vi "doT1.vi"(8 "q_samples":i32=50, 10 "parameters_recenter":T5={"input_xyz"={"X_um"=0.0, "Y_um"=0.0, "Z_um"=0.0}, "recenter"=FALSE, "recenter_s"=3}, 11 "Rabi_parameters":T6) -> (0 "triggers":u32[][](array[numeric]), 1 "std_deviation":dbl[](array[numeric]), 2 "Rabi_curve":cluster{dbl[], "dark_time_us":dbl[]}(graph), 3 "timetags":u32[][](array[numeric]), 5 "position_xyzt":T1, 7 "mini_scan":T2)   [LabVIEW 2018]
uses:
  <vilib>/Analysis/NI_AALBase.lvlib
panel:
  in  "parameters_z-scan":T3={"dwell_time_ms"=2.0, "q_steps"=5, "span_um"=1.0, "refocus"=TRUE}
  in  "parameters_xy-scan":T4={"image_size_xy_um"=2.0, "frame_size_xy_px"=7, "dwell_time_ms"=0.5}
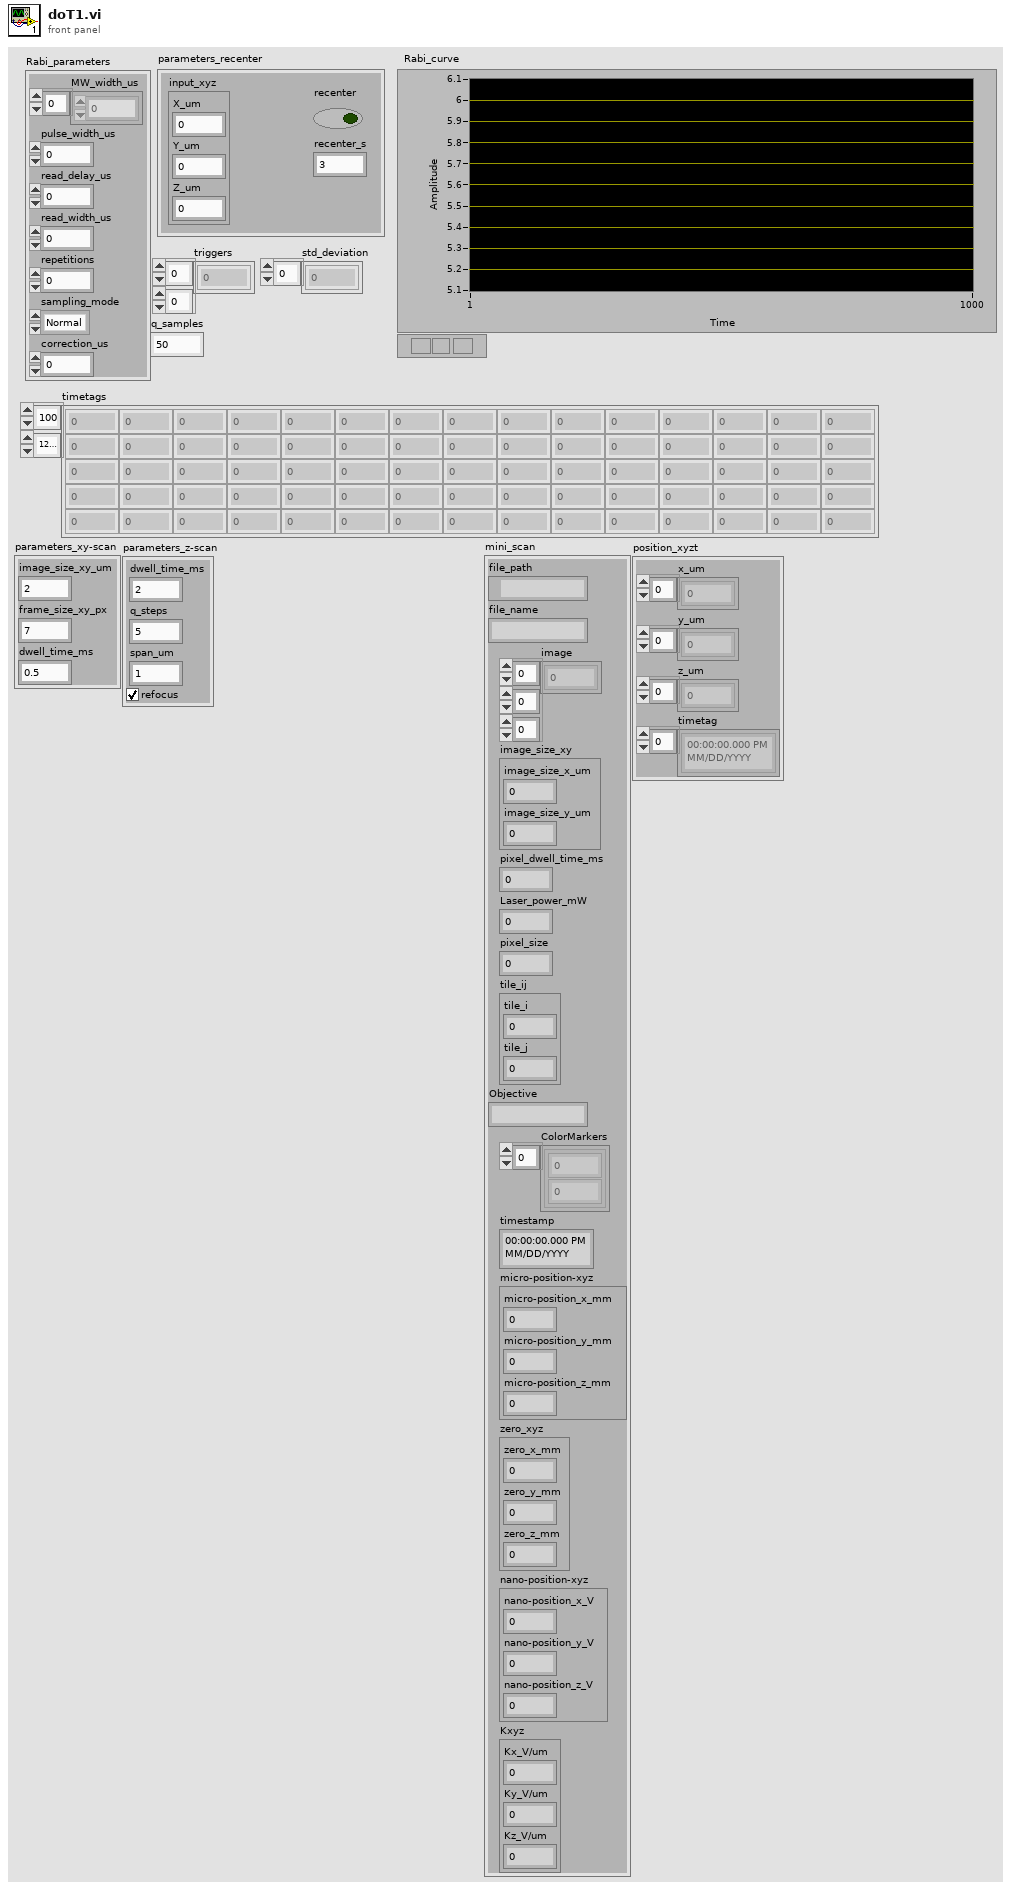
[diagram p1: front panel]
types:
  T1 = cluster{"x_um":sgl[], "y_um":sgl[], "z_um":sgl[], "timetag":timestamp[]}
  T2 = cluster{"file_path":path, "file_name":string, "image":dbl[][][], "image_size_xy":cluster{"image_size_x_um":sgl, "image_size_y_um":sgl}, "pixel_dwell_time_ms":sgl, "Laser_power_mW":sgl, "pixel_size":dbl, "tile_ij":cluster{"tile_i":i32, "tile_j":i32}, "Objective":string, "ColorMarkers":cluster{dbl, u32}[], "timestamp":timestamp, "micro-position-xyz":cluster{"micro-position_x_mm":sgl, "micro-position_y_mm":sgl, "micro-position_z_mm":sgl}, "zero_xyz":cluster{"zero_x_mm":dbl, "zero_y_mm":dbl, "zero_z_mm":dbl}, "nano-position-xyz":cluster{"nano-position_x_V":sgl, "nano-position_y_V":sgl, "nano-position_z_V":sgl}, "Kxyz":cluster{"Kx_V/um":sgl, "Ky_V/um":sgl, "Kz_V/um":sgl}}
  T3 = cluster{"dwell_time_ms":dbl, "q_steps":u32, "span_um":dbl, "refocus":bool}
  T4 = cluster{"image_size_xy_um":dbl, "frame_size_xy_px":u32, "dwell_time_ms":dbl}
  T5 = cluster{"input_xyz":cluster{"X_um":sgl, "Y_um":sgl, "Z_um":sgl}, "recenter":bool, "recenter_s":u32}
  T6 = cluster{"MW_width_us":dbl[], "pulse_width_us":dbl, "read_delay_us":dbl, "read_width_us":dbl, "repetitions":i32, "sampling_mode":enum16{"Normal", "Sweep"}, "correction_us":dbl}
  T7 = cluster{"Instruct Data":i32, "Op Code":i32, "Flags":bool[], "Comments":string, "Time":dbl}[]
  T8 = cluster{"nano-position_X_um":sgl, "nano-position_Y_um":sgl, "nano-position Z_um":sgl}
  T9 = cluster{"nano-position_X_um":sgl, "nano-position_Y_um":sgl, "nano-position Z_um":sgl}[]
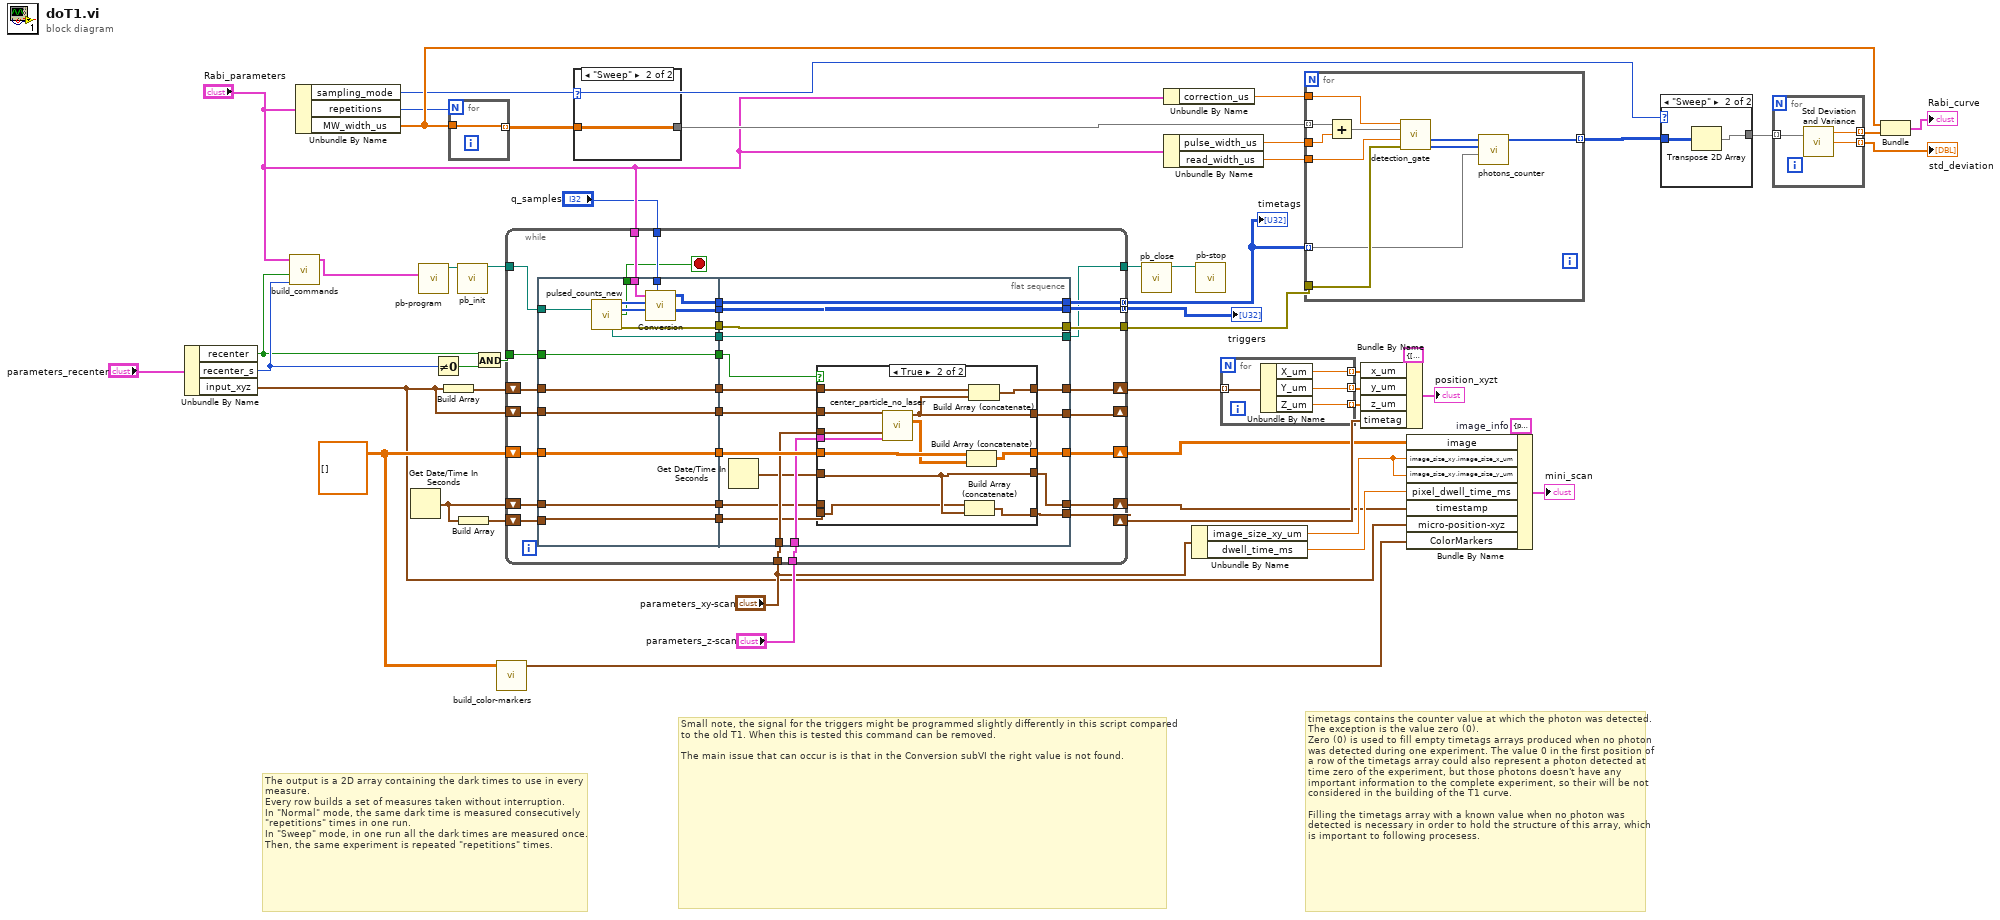
[diagram p0: block diagram]
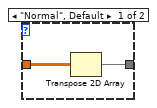
[diagram p3: hidden frame]
diagram:
  w20 = T2 {"file_path"=path "", "file_name"="", "image"=[], "image_size_xy"={"image_size_x_um"=1.0, "image_size_y_um"=1.0}, "pixel_dwell_time_ms"=1.0, "Laser_power_mW"=1.0, "pixel_size"=0.0, "tile_ij"={"tile_i"=0, "tile_j"=0}, "Objective"="", "ColorMarkers"=[], "timestamp"=timestamp(0 s since 1904-01-01), "micro-position-xyz"={"micro-position_x_mm"=1.0, "micro-position_y_mm"=1.0, "micro-position_z_mm"=1.0}, "zero_xyz"={"zero_x_mm"=0.0, "zero_y_mm"=0.0, "zero_z_mm"=0.0}, "nano-position-xyz"={"nano-position_x_V"=1.0, "nano-position_y_V"=1.0, "nano-position_z_V"=1.0}, "Kxyz"={"Kx_V/um"=1.0, "Ky_V/um"=1.0, "Kz_V/um"=1.0}}  # image_info
  w31 = dbl[][][] []
  # "Small note, the signal for the triggers might be programmed slightly differently in this script compared to the old T1. When this is tested this command can be removed.\n\nThe main issue that can occur is is that in the Conversion subVI the right value is not found."
  # "timetags contains the counter value at which the photon was detected. The exception is the value zero (0).\nZero (0) is used to fill empty timetags arrays produced when no photon was detected during one experiment. The value 0 in the first position of a row of the timetags array could also represent a photon detected at time zero of the experiment, but those photons doesn't have any important information to the complete experiment, so their will be not considered in the building of the T1 curve.\n\nFilling the timetags array with a known value when no photon was detected is necessary in order to hold the structure of this array, which is important to following procesess."
  # "The output is a 2D array containing the dark times to use in every measure.\nEvery row builds a set of measures taken without interruption.\nIn \"Normal\" mode, the same dark time is measured consecutively \"repetitions\" times in one run.\nIn \"Sweep\" mode, in one run all the dark times are measured once. Then, the same experiment is repeated \"repetitions\" times."
  n1 = Unbundle By Name("parameters_recenter") -> ("recenter"=w11:bool, "recenter_s"=w33:u32, "input_xyz"=w15:cluster{"X_um":sgl, "Y_um":sgl, "Z_um":sgl})
  n2 = call "build_commands.vi"("Refocus_s"=w33, "Refocus?"=w11, "T1_parameters"="Rabi_parameters") -> ("instructions_array"=w4:T7)  [unwired: 8 in]
  n3 = Unbundle By Name("Rabi_parameters") -> ("sampling_mode"=w40:enum16{"Normal", "Sweep"}, "repetitions"=w9:i32, "MW_width_us"=w41:dbl[])
  n4 = Get Date/Time In Seconds() -> (seconds since 1Jan1904=w28:timestamp)
  n5 = call "pb-program.vi"("Commands"=w4) -> ("path out"=w3:path)  [unwired: 10 in]
  n6 = Not Equal To 0?(x=w33) -> (x != 0?=w34:bool)
  n7 = Build Array(w15) -> (w35:cluster{"X_um":sgl, "Y_um":sgl, "Z_um":sgl}[])
  n8 = for {
    N: w9 -> [_]
    tunnel: [w50] -> w39 mode=indexing
    tunnel: w41 -> [w50]
  }
  n9 = call "pb_init.vi"("path in"=w3) -> ("path out"=w5:path)  [unwired: 9 in, 1 out]
  n10 = Build Array(w28) -> (w29:timestamp[])
  n11 = And(x=w11, y=w34) -> (x .and. y?=w32:bool)
  n12 = call "build_color-markers.vi"("images"=w31) -> ("color_markers"=w14:cluster{dbl, u32}[])  [unwired: 10 in]
  n13 = while {
    tunnel: [w81] -> w36
    tunnel: [w80] -> w12 mode=concatenating
    tunnel: [w79] -> w13 mode=concatenating
    shift-right: [w68] -> w27
    shift-left: w35 -> [w75]
    tunnel: w32 -> [w72]
    shift-right: [w69] -> _
    shift-left: w15 -> [w71]
    shift-right: [w57] -> w19
    shift-left: w31 -> [w67]
    tunnel: "parameters_xy-scan" -> [w65]
    tunnel: "parameters_z-scan" -> [w64]
    shift-right: [w58] -> w22
    shift-left: w29 -> [w63]
    shift-right: [w62] -> w16
    shift-left: w28 -> [w61]
    tunnel: "Rabi_parameters" -> [w56]
    tunnel: "q_samples" -> [w55]
    tunnel: w5 -> [w53]
    tunnel: [w51] -> w7
    stop <- w54 stop-if-true
    n14 = flat-sequence {
      tunnel: [w97] -> w78
      tunnel: [w90] -> w77
      tunnel: [w89] -> w76
      tunnel: w75 -> [w96]
      tunnel: [w96] -> w74
      tunnel: [w95] -> w73
      tunnel: w72 -> [w95]
      tunnel: w71 -> [w94]
      tunnel: [w94] -> w70
      tunnel: w67 -> [w93]
      tunnel: [w93] -> w66
      tunnel: w63 -> [w91]
      tunnel: w61 -> [w92]
      tunnel: [w92] -> w60
      tunnel: [w91] -> w59
      tunnel: w56 -> [w88]
      tunnel: w55 -> [w85]
      tunnel: [w84] -> w54
      tunnel: w53 -> [w83]
      tunnel: [w82] -> w52
      tunnel: [w113] -> w79
      tunnel: [w114] -> w80
      tunnel: [w115] -> w81
      tunnel: w78 -> [w115]
      tunnel: w77 -> [w114]
      tunnel: w76 -> [w113]
      tunnel: w74 -> [w112]
      tunnel: w73 -> [w98]
      tunnel: w70 -> [w111]
      tunnel: [w110] -> w69
      tunnel: [w109] -> w68
      tunnel: w66 -> [w108]
      tunnel: w65 -> [w107]
      tunnel: w64 -> [w106]
      tunnel: [w104] -> w62
      tunnel: w60 -> [w103]
      tunnel: w59 -> [w102]
      tunnel: [w101] -> w58
      tunnel: [w100] -> w57
      tunnel: w52 -> [w99]
      tunnel: [w99] -> w51
      frame #0 {
        n15 = call "pulsed_counts_new.vi"("path in"=w83) -> ("timetags"=w87:u32[], "triggers"=w86:u32[], "stop measure"=w84:bool, "path out"=w82:path, "Error_out"=w97:errorcluster)  [unwired: 10 in]
        n16 = call "Conversion.vi"("q_samples"=w85, "triggers"=w86, "timetags"=w87, "Rabi_parameters"=w88) -> ("triggers"=w90:u32[][], "timetags"=w89:u32[][])  [unwired: 6 in]
      }
      frame #1 {
        n17 = Get Date/Time In Seconds() -> (seconds since 1Jan1904=w105:timestamp)
        n18 = case shown="True" w98 {
          tunnel: w112 -> [w120 w132]
          tunnel: w111 -> [w119 w131]
          tunnel: [w119 w130] -> w110
          tunnel: [w120 w129] -> w109
          tunnel: w108 -> [w116 w128]
          tunnel: w107 -> [_ w126]
          tunnel: w106 -> [_ w125]
          tunnel: w105 -> [_ w124]
          tunnel: [w118 w124] -> w104
          tunnel: w103 -> [w118 _]
          tunnel: w102 -> [w117 w123]
          tunnel: [w117 w122] -> w101
          tunnel: [w116 w121] -> w100
          frame False {
          }
          frame True {
            n19 = call "center_particle_no_laser.vi"("input_xyz"=w131, "parameters_xy-scan"=w126, "parameters_z-scan"=w125) -> ("output_xyz"=w130:T8, "mini_scan"=w127:dbl[][])  [unwired: 11 in]
            n20 = Build Array (concatenate)(w123, w124) -> (w122:timestamp[])
            n21 = Build Array (concatenate)(w128, w127) -> (w121:dbl[][][])
            n22 = Build Array (concatenate)(w132, w130) -> (w129:T9)
          }
        }
      }
    }
  }
  "timetags" <- w13
  "triggers" <- w12
  n23 = case shown="\"Sweep\"" w40 {
    tunnel: w39 -> [w134 w135]
    tunnel: [w133 w135] -> w38
    frame "Normal", Default {
      n24 = Transpose 2D Array(2D array=w134) -> (transposed array=w133:dbl[][])
    }
    frame "Sweep" {
    }
  }
  n25 = call "pb_close.vi"("path in"=w7) -> ("path out"=w6:path)  [unwired: 9 in, 1 out]
  n26 = Unbundle By Name("Rabi_parameters") -> ("correction_us"=w43:dbl)
  n27 = Unbundle By Name("Rabi_parameters") -> ("pulse_width_us"=w42:dbl, "read_width_us"=w44:dbl)
  n28 = Unbundle By Name("parameters_xy-scan") -> ("image_size_xy_um"=w18:dbl, "dwell_time_ms"=w17:dbl)
  n29 = call "pb-stop.vi"("path in"=w6) -> ()  [unwired: 9 in, 2 out]
  n30 = for {
    tunnel: w27 -> [w139] mode=indexing
    tunnel: [w138] -> w25 mode=indexing
    tunnel: [w137] -> w24 mode=indexing
    tunnel: [w136] -> w23 mode=indexing
    n31 = Unbundle By Name(w139) -> ("X_um"=w138:sgl, "Y_um"=w137:sgl, "Z_um"=w136:sgl)
  }
  n32 = for {
    tunnel: [w149] -> w45 mode=indexing
    tunnel: w44 -> [w148]
    tunnel: w36 -> [w147]
    tunnel: w43 -> [w144]
    tunnel: w42 -> [w143]
    tunnel: w38 -> [w141] mode=indexing
    tunnel: w13 -> [w140] mode=indexing
    n33 = Add(x=w141, y=w143) -> (x+y=w142:dbl[])
    n34 = call "detection_gate.vi"("Error_in"=w147, "read_width_us"=w148, "pulse_period_us"=w142, "correction_us"=w144) -> ("start_read"=w145:u32[], "stop_read"=w146:u32[])  [unwired: 6 in]
    n35 = call "photons_counter.vi"("timetags"=w140, "start_read"=w145, "stop_read"=w146) -> ("photons_counts"=w149:i32[])  [unwired: 8 in]
  }
  n36 = Bundle By Name(cluster=T1 {"x_um"=[], "y_um"=[], "z_um"=[], "timetag"=[]} ("position_xyzt"), "x_um"=w25, "y_um"=w24, "z_um"=w23, "timetag"=w22) -> (→"position_xyzt":T1)
  n37 = Bundle By Name(cluster=w20, "image"=w19, "image_size_xy.image_size_x_um"=w18, "image_size_xy.image_size_y_um"=w18, "pixel_dwell_time_ms"=w17, "timestamp"=w16, "micro-position-xyz"=w15, "ColorMarkers"=w14) -> (→"mini_scan":T2)
  n38 = case shown="\"Sweep\"" w40 {
    tunnel: w45 -> [w150 w152]
    tunnel: [w150 w151] -> w48
    frame "Normal", Default {
    }
    frame "Sweep" {
      n39 = Transpose 2D Array(2D array=w152) -> (transposed array=w151:i32[][])
    }
  }
  n40 = for {
    tunnel: w48 -> [w155] mode=indexing
    tunnel: [w154] -> w47 mode=indexing
    tunnel: [w153] -> w46 mode=indexing
    n41 = call <vilib>:"Std Deviation and Variance.vi"("X"=w155) -> ("mean"=w154:dbl, "standard deviation"=w153:dbl)  [unwired: 1 in, 1 out]
  }
  "std_deviation" <- w46
  n42 = Bundle("MW_width_us"=w41, w47) -> (→"Rabi_curve":cluster{"MW_width_us":dbl[], dbl[]})  [unwired: 1 in]
